vi "Destroy User Events.vi"(8 "error in":errorcluster, 11 "Optimization in":refnum<class "Optimization.lvclass">) -> (0 "error out":errorcluster, 3 "Optimization out":refnum<class "Optimization.lvclass">)   [LabVIEW 2016, in "Optimization Framework.lvlib" / "Optimization.lvclass"]
uses:
  Optimization.lvclass
  Optimization.lvclass/Optimization.ctl
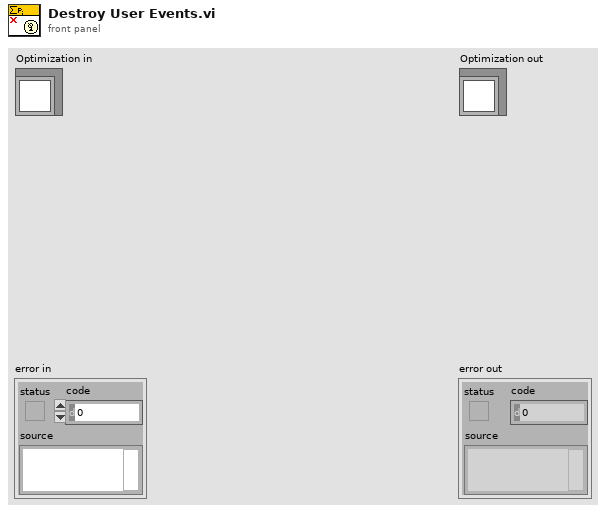
[diagram p1: front panel]
types:
  T1 = typedef "Optimization Framework.lvlib/Optimization.lvclass/Optimization User Events.ctl" = cluster{"Microgrid State":refnum<user-event>, "stop":refnum<user-event>}
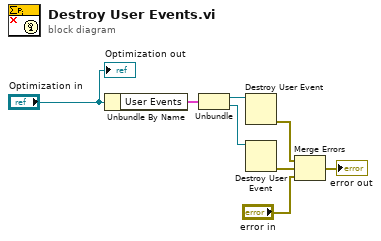
[diagram p0: block diagram]
diagram:
  n1 = Unbundle By Name("Optimization in") -> ("User Events"=w5:T1)
  n2 = Unbundle(w5) -> ("Microgrid State"=w4:refnum<user-event>, "stop"=w2:refnum<user-event>)
  n3 = Destroy User Event(user event=w4) -> (error out=w3:errorcluster)  [unwired: 1 in]
  n4 = Destroy User Event(user event=w2) -> (error out=w1:errorcluster)  [unwired: 1 in]
  n5 = Merge Errors(w3, w1, "error in") -> (→"error out":errorcluster)
  "Optimization out" <- "Optimization in"
